vi "VelocityCalculator.vi"(8 "Offset (V)":dbl, 11 "Voltage Input":dbl[](array[numeric])) -> (3 "Veloctiy Output [m/s]":dbl[](array[numeric]))   [LabVIEW 2017]
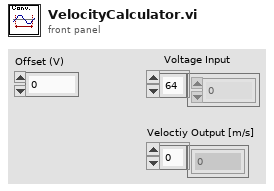
[diagram p1: front panel]
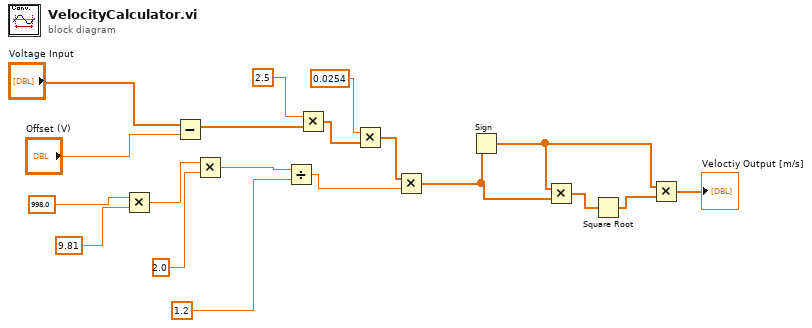
[diagram p0: block diagram]
diagram:
  n1 = Multiply(x=998.0, y=9.81) -> (x*y=w10:dbl)
  n2 = Subtract(x="Voltage Input", y="Offset (V)") -> (x-y=w5:dbl[])
  n3 = Multiply(x=w10, y=2.0) -> (x*y=w12:dbl)
  n4 = Divide(x=w12, y=1.2) -> (x/y=w4:dbl)
  n5 = Multiply(x=2.5, y=w5) -> (x*y=w2:dbl[])
  n6 = Multiply(x=0.0254, y=w2) -> (x*y=w1:dbl[])
  n7 = Multiply(x=w1, y=w4) -> (x*y=w17:dbl[])
  n8 = Sign(1:w17) -> (0:w14:dbl[])
  n9 = Multiply(x=w14, y=w17) -> (x*y=w16:dbl[])
  n10 = Square Root(x=w16) -> (sqrt(x)=w13:dbl[])
  n11 = Multiply(x=w14, y=w13) -> (x*y=→"Veloctiy Output [m/s]":dbl[])
